vi "launch_test_1.vi"(8 "error in (no error)":errorcluster, 9 "Message Queues in":T2, 11 "test mode":T1(ring)) -> (0 "error out":errorcluster)   [LabVIEW 2015]
uses:
  support/Message Queue/All Message Queues.ctl
  support/Message Queue/Message Cluster.ctl
  support/Message Queue/Enqueue Message (Array).vi
  support/Message Queue/Message Queue.lvlib
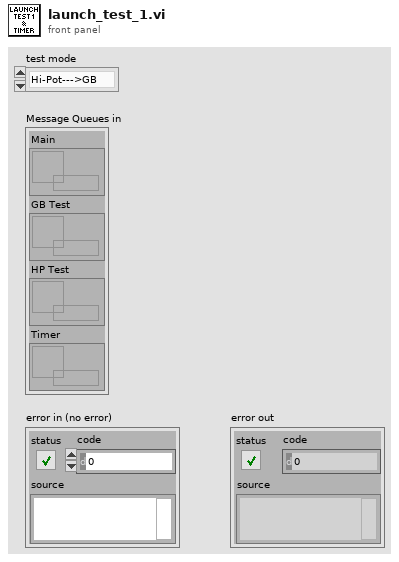
[diagram p1: front panel]
types:
  T1 = enum16{"Hi-Pot--->GB", "GB--->Hi-Pot", "Hi-Pot only", "GB only"}
  T2 = typedef "Message Queue.lvlib/All Message Queues.ctl" = cluster{"Main":refnum<queue>, "GB Test":refnum<queue>, "HP Test":refnum<queue>, "Timer":refnum<queue>}
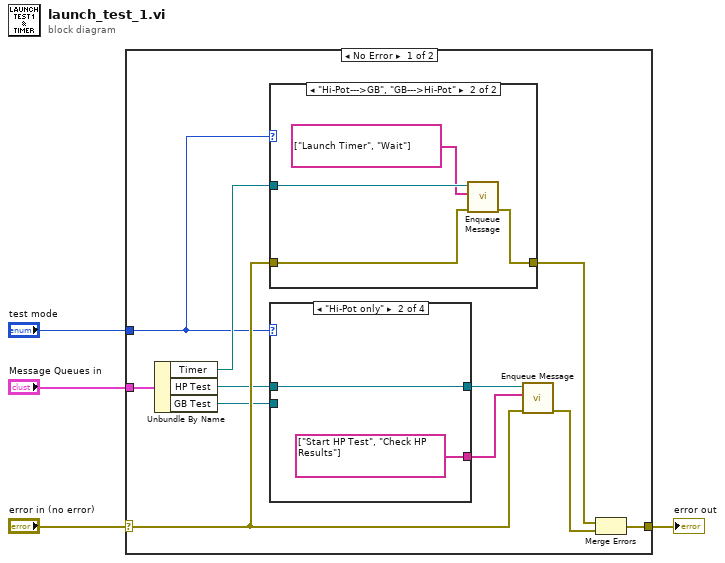
[diagram p0: block diagram]
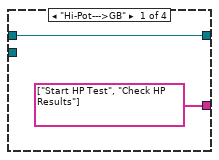
[diagram p3: hidden frame]
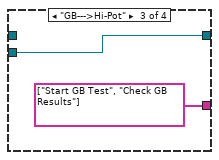
[diagram p4: hidden frame]
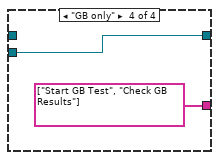
[diagram p5: hidden frame]
diagram:
  n1 = case shown="No Error" "error in (no error)" {
    selector: "error in (no error)" -> [w15 w29]
    tunnel: "Message Queues in" -> [w12 _]
    tunnel: "test mode" -> [w7 _]
    tunnel: [w6 w29] -> w1
    frame No Error {
      n2 = Unbundle By Name(w12) -> ("Timer"=w8:refnum<queue>, "HP Test"=w13:refnum<queue>, "GB Test"=w14:refnum<queue>)
      n3 = case shown="\"Hi-Pot--->GB\", \"GB--->Hi-Pot\"" w7 {
        tunnel: [w16 w20] -> w5
        tunnel: w15 -> [w16 w19]
        tunnel: w8 -> [_ w18]
        frame "Hi-Pot only", "GB only" {
        }
        frame "Hi-Pot--->GB", "GB--->Hi-Pot" {
          n4 = call-poly "Enqueue Message.vi"("error in (no error)"=w19, "Message Array"=string[] ["Launch Timer", "Wait"], "Message Queue"=w18) -> ("error out"=w20:errorcluster)  [unwired: 7 in, 1 out]
        }
      }
      n5 = case shown="\"Hi-Pot only\"" w7 {
        tunnel: w13 -> [w22 w23 _ _]
        tunnel: [w22 w23 w25 w27] -> w11
        tunnel: [string[] ["Start HP Test", "Check HP Results"] string[] ["Start HP Test", "Check HP Results"] string[] ["Start GB Test", "Check GB Results"] string[] ["Start GB Test", "Check GB Results"]] -> w10
        tunnel: w14 -> [_ _ w25 w27]
        frame "Hi-Pot--->GB" {
        }
        frame "Hi-Pot only" {
        }
        frame "GB--->Hi-Pot" {
        }
        frame "GB only" {
        }
      }
      n6 = call-poly "Enqueue Message.vi"("error in (no error)"=w15, "Message Array"=w10, "Message Queue"=w11) -> ("error out"=w9:errorcluster)  [unwired: 7 in, 1 out]
      n7 = Merge Errors(w5, w9) -> (w6:errorcluster)
    }
    frame Error {
    }
  }
  "error out" <- w1
